vi "OOB Performance Test Channel.vi"() -> ()   [LabVIEW 2021]
uses:
  <vilib>/Platform/TimedLoop/XDataNode/timing_clust.ctl
  <vilib>/Platform/TimedLoop/XDataNode/nitl_modes.ctl
  <vilib>/Platform/TimedLoop/XDataNode/wakeup.ctl
  CIFOutOfBand.lvclass/CIFOutOfBand.ctl
  ecd22e40-9ef3-47c9-84dd-6e51471c5b7d.vi
  cc845de9-9662-4d69-8494-93190ebbf16f.vi
  5dde9a10-7574-45f3-be33-437a2b751792.vi
  630e717b-411c-4f0a-96f3-098c02e0b307.vi
  27ef35cb-55c2-4e73-bad1-dda663d636b9.vi
  ecd22e40-9ef3-47c9-84dd-6e51471c5b7d.vi/c28b0ead-42ad-4072-80a2-aca7f2bd7ce3.vi
  cc845de9-9662-4d69-8494-93190ebbf16f.vi/4bc1c15b-36ab-481f-b8dd-c64075ce723a.vi
  cc845de9-9662-4d69-8494-93190ebbf16f.vi/d83cb72b-7713-41fc-a3d1-682de79cf574.vi
  5dde9a10-7574-45f3-be33-437a2b751792.vi/c28b0ead-42ad-4072-80a2-aca7f2bd7ce3.vi
  630e717b-411c-4f0a-96f3-098c02e0b307.vi/c28b0ead-42ad-4072-80a2-aca7f2bd7ce3.vi
  630e717b-411c-4f0a-96f3-098c02e0b307.vi/219d0231-d98b-4193-b5cc-84f90e3c9091.vi
  27ef35cb-55c2-4e73-bad1-dda663d636b9.vi/c28b0ead-42ad-4072-80a2-aca7f2bd7ce3.vi
  27ef35cb-55c2-4e73-bad1-dda663d636b9.vi/219d0231-d98b-4193-b5cc-84f90e3c9091.vi
  CIF-Core-LabVIEW/src/CIFServices/CIFServices Fill In Error Info Ex.vi
  CIFOutOfBand.lvclass
  <vilib>/Platform/TimedLoop/XDataNode/XDataNode.xnode
  <vilib>/Platform/TimedLoop/XDataNode/XDNodeRunTimeDep.lvlib
  CIF-Core-LabVIEW/src/CIFServices/CifChannelServices.lvlib
panel:
  out "avg no unflat":dbl
  out "Max no unflat":dbl
  out "channel":dbl
  out "channel":dbl
  out "avg no conflict":dbl
  out "Max no conflict":dbl
  out "avg simple":dbl
  out "Max simple":dbl
  out "Max Complex":dbl
  out "avg complex":dbl
  out "pass":bool
  out "error out":errorcluster
  # "This test should be run on RT.  It stresses the communications by constantly creating resource contraints with the low priority sender and the high priority loop. On Windows the priority of the loops cannot be set."
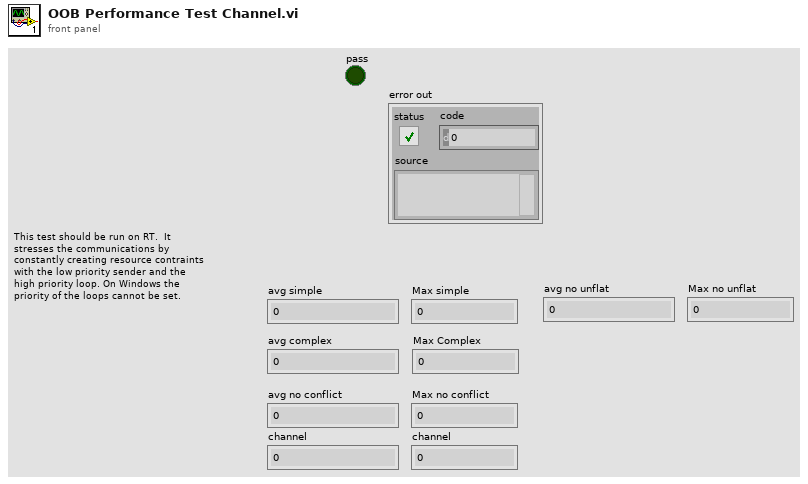
[diagram p1: front panel]
types:
  T1 = typedef "XDNodeRunTimeDep.lvlib/timing_clust.ctl" = cluster{"Expected End [f-1]":u64, "Actual End [f-1]":u64, "Finished Late? [f-1]":bool, "Expected End [i-1]":u64, "Actual End [i-1]":u64, "Finished Late? [i-1]":bool, "Expected Start [i]":u64, "Actual Start [i]":u64, "Expected Start [f]":u64, "Actual Start [f]":u64, "Source Name":string, "Structure Name":string, "Period":i64, "Deadline":i64, "Offset":i64, "Start":i64, "Priority":i32, "Timeout":i32, "Mode":T2, "Wakeup Reason":T3, "Error":errorcluster, "Source Type":string, "Secondary Source Type":string, "Global End Time":u64, "Global Start Time":u64, "Frame Duration":u64, "Iteration Duration":u64, "Assigned CPU":i32, "I/O Scan Engine Mode":u32}
  T2 = typedef "XDNodeRunTimeDep.lvlib/nitl_modes.ctl" = enum32{"No Change", "Process missed periods, maintain original phase", "Discard missed periods, maintain original phase", "Process missed periods, ignore original phase", "Discard missed periods, ignore original phase"}
  T3 = typedef "XDNodeRunTimeDep.lvlib/wakeup.ctl" = enum32{"Normal", "Aborted", "Asynchronous wakeup", "Timing source error", "Timed loop error", "Timeout"}
  T4 = cluster{"Numeric":dbl, "Array":cluster{"Numeric":dbl, "String":string, "Boolean":bool}[], "string":string, "Null array":u8[]}
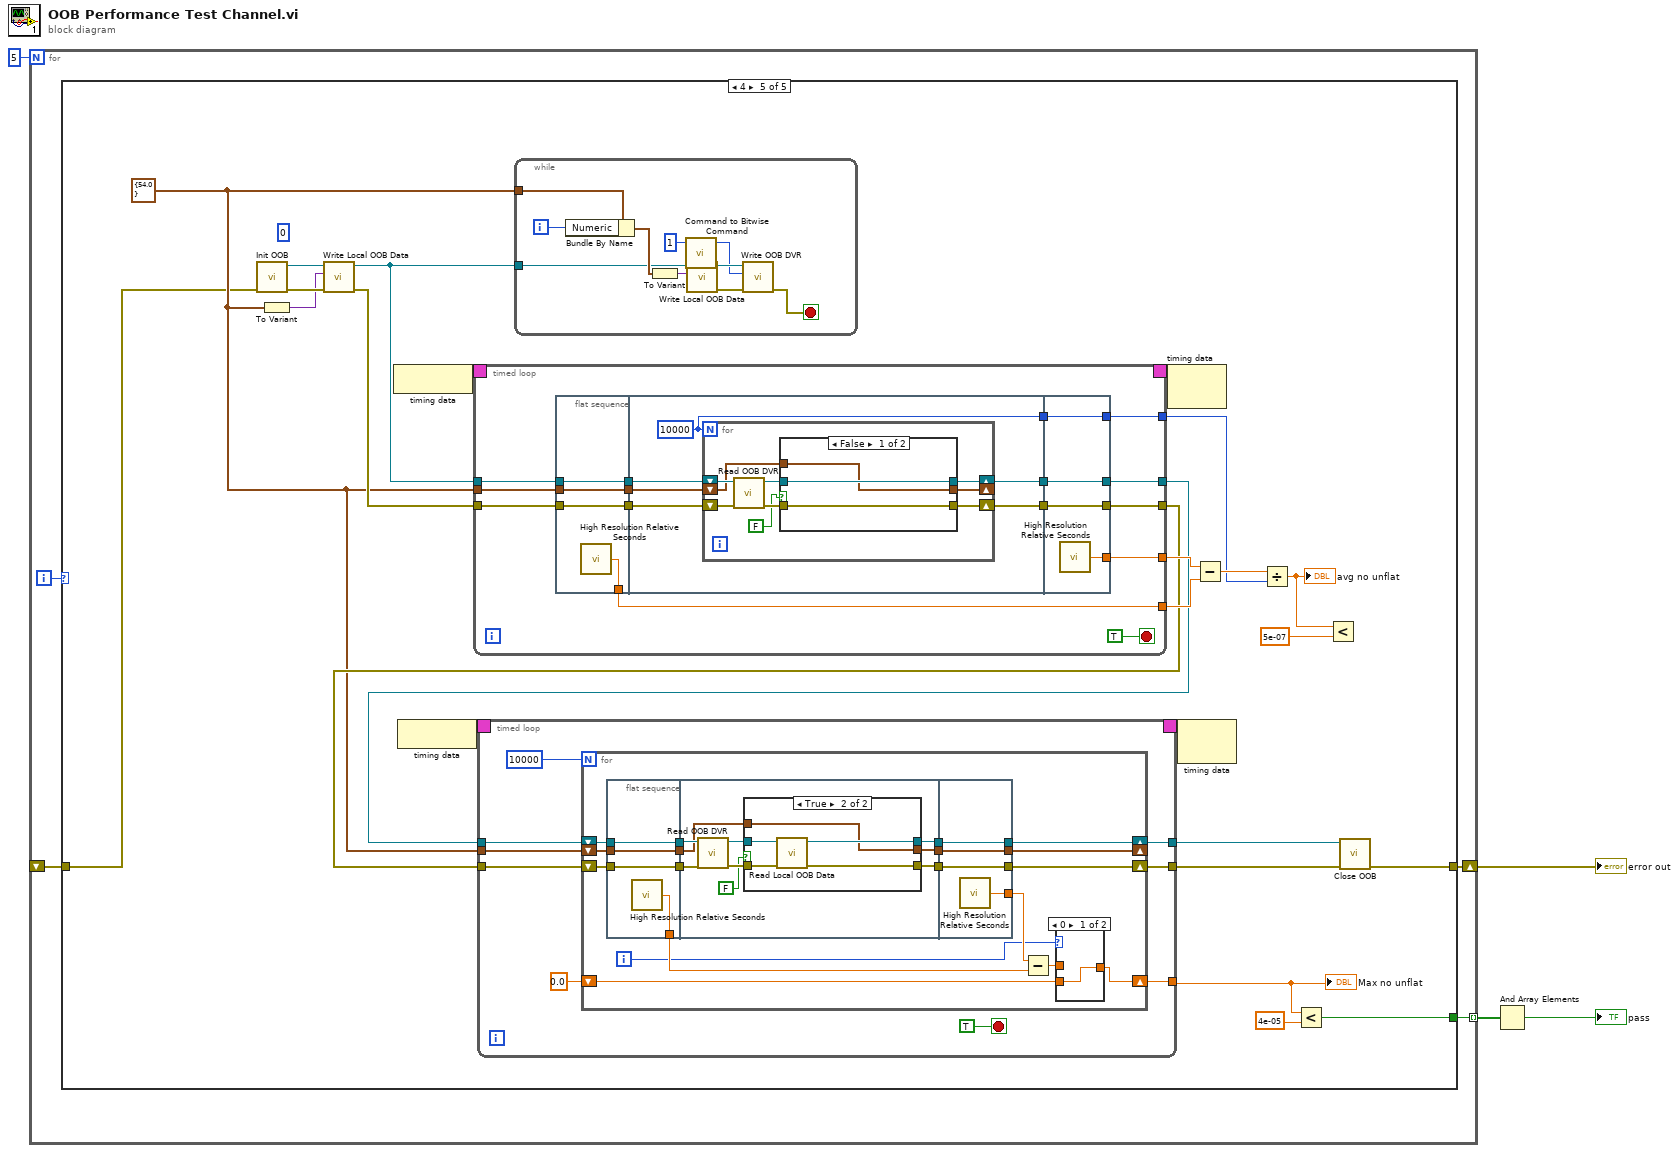
[diagram p0: block diagram]
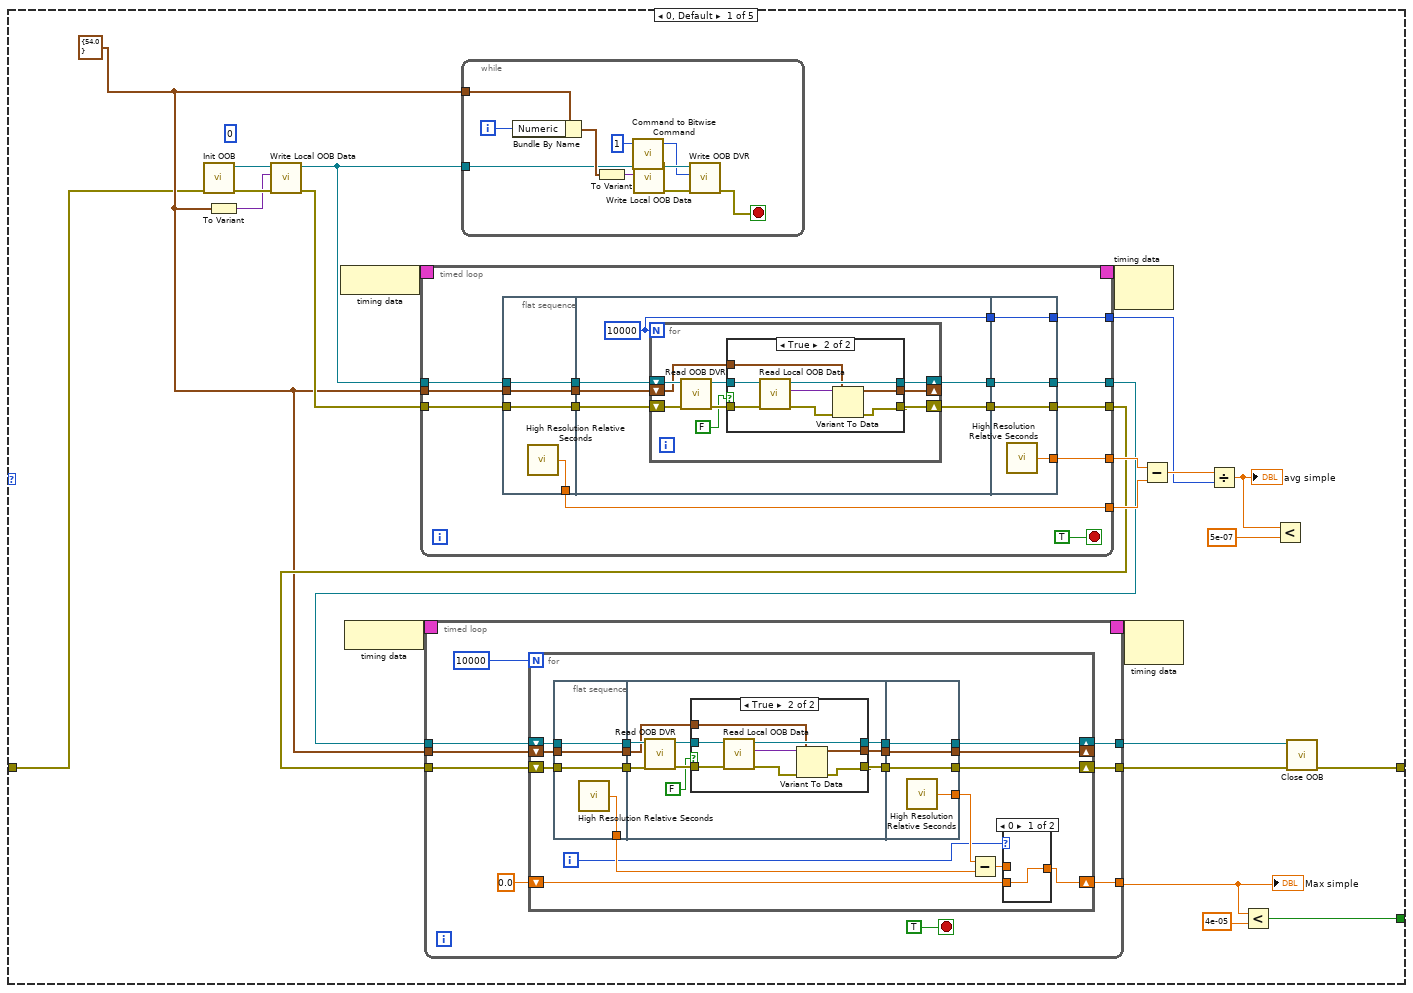
[diagram p2: hidden frame]
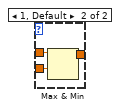
[diagram p3: hidden frame]
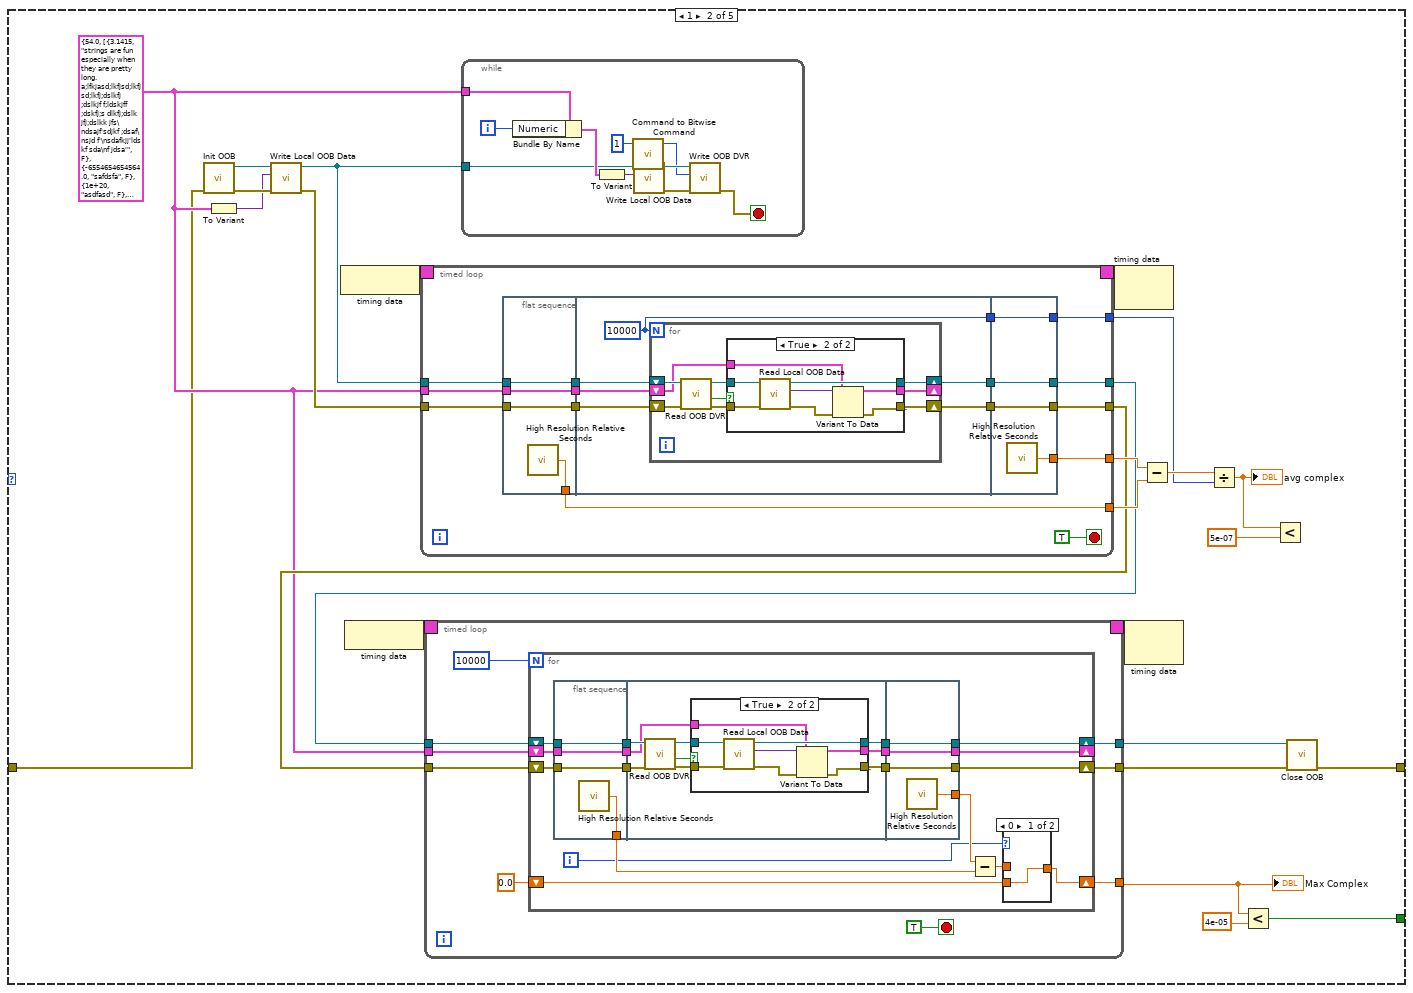
[diagram p6: hidden frame]
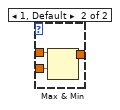
[diagram p7: hidden frame]
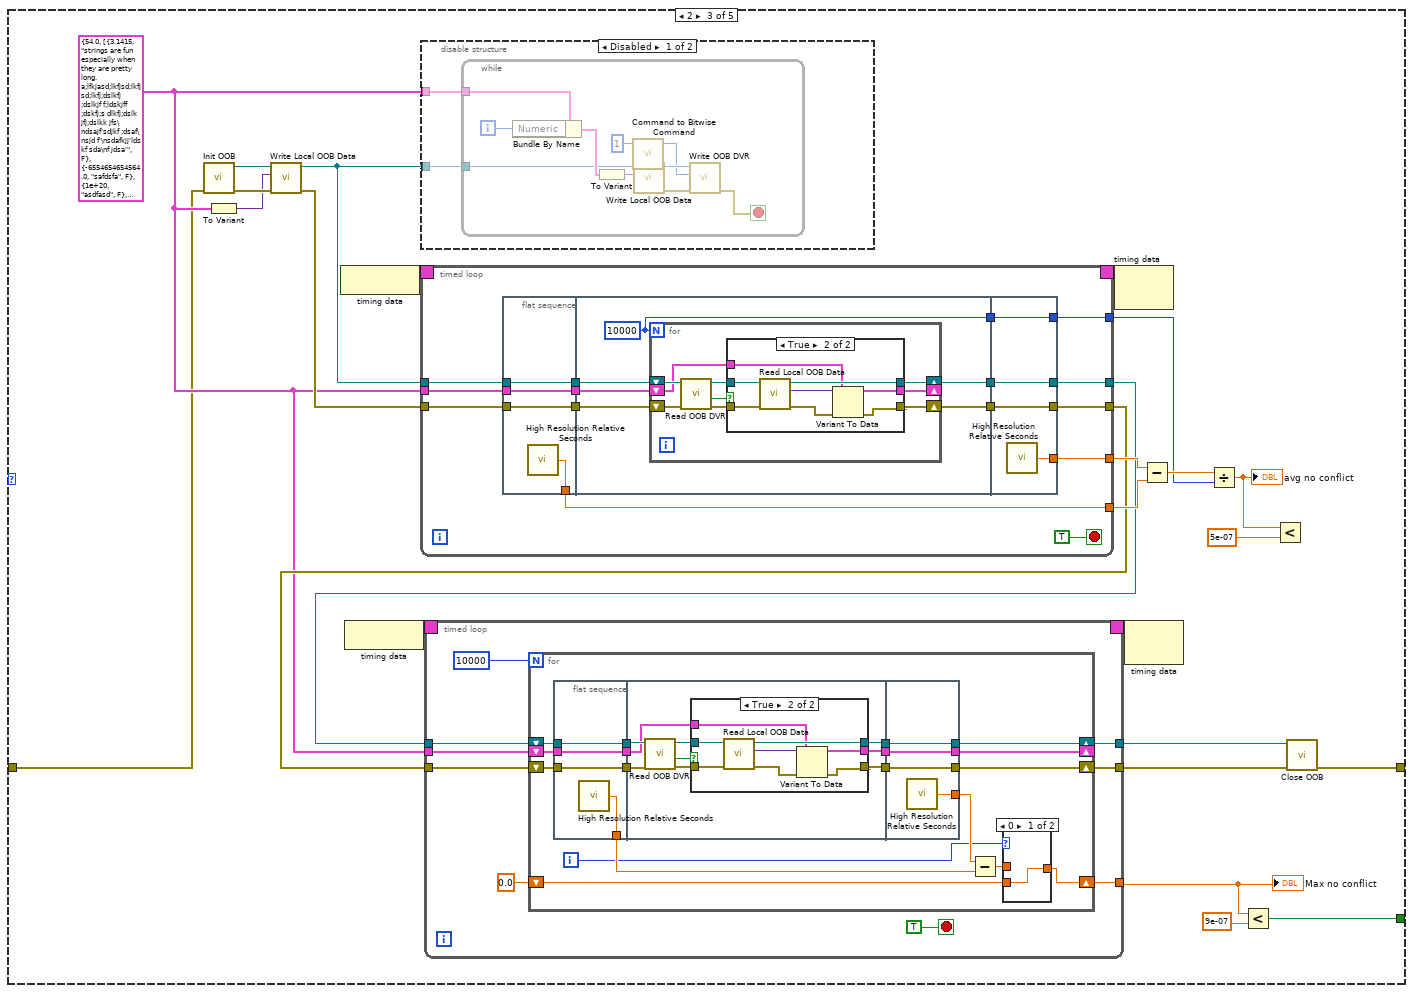
[diagram p10: hidden frame]
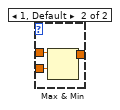
[diagram p12: hidden frame]
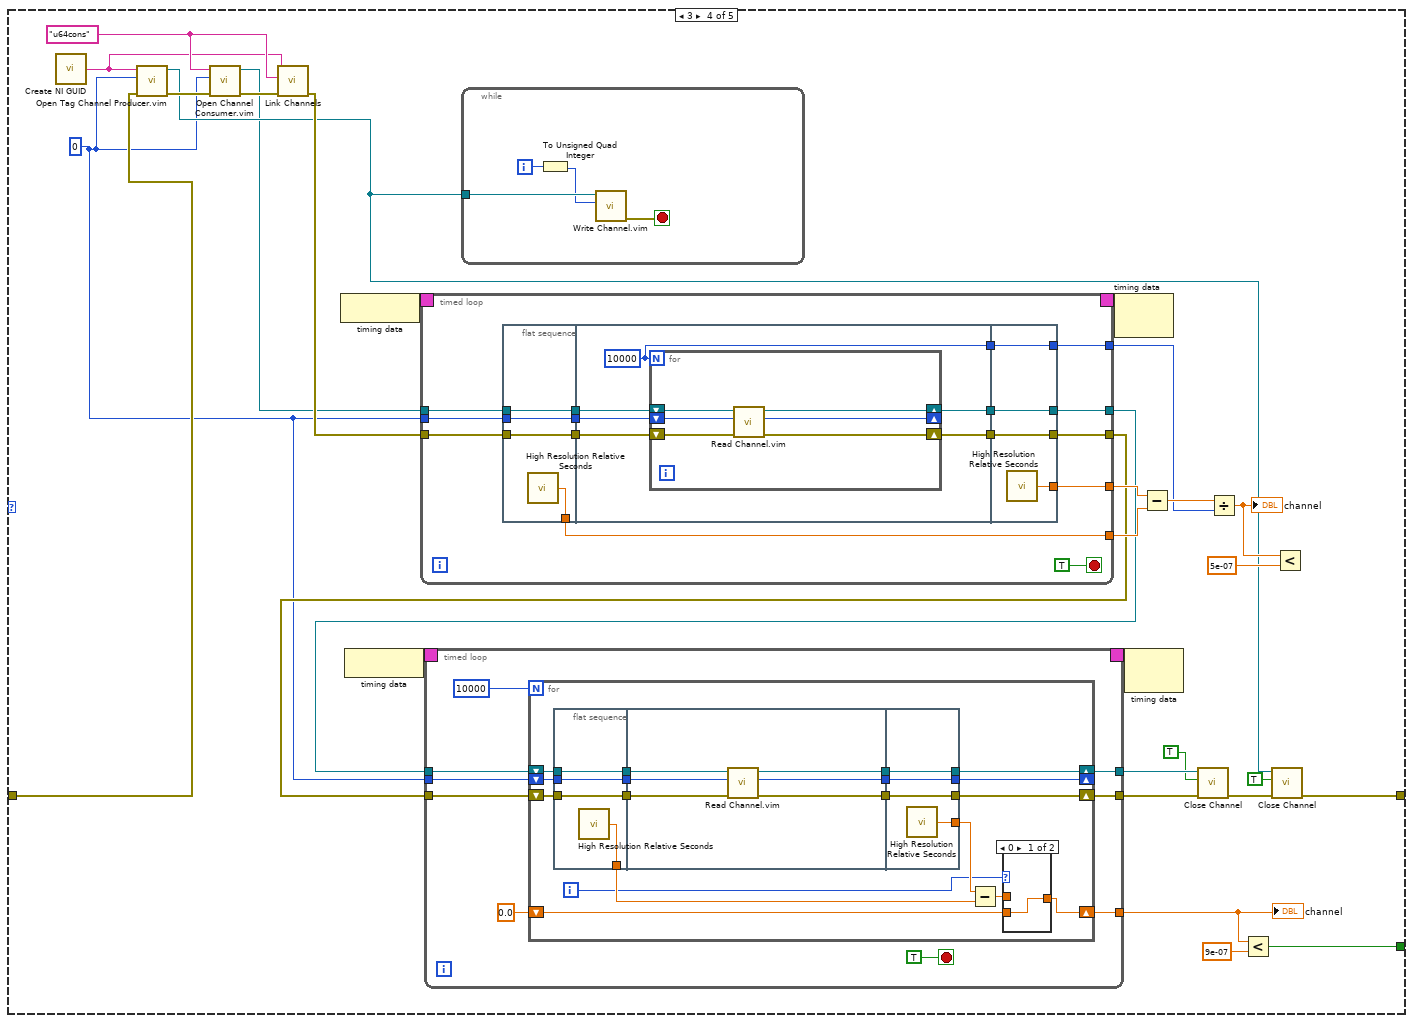
[diagram p15: hidden frame]
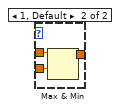
[diagram p16: hidden frame]
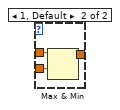
[diagram p17: hidden frame]
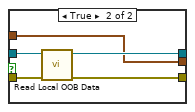
[diagram p19: hidden frame]
diagram:
  n1 = for {
    N: 5 -> [_]
    tunnel: [w8] -> w2 mode=indexing
    shift-right: [w7] -> w4
    shift-left: _ -> [w5]
    i -> [w6]
    n2 = case shown="4" w6 {
      tunnel: [w19 w168 w317 w473 w590] -> w8
      tunnel: [w16 w165 w314 w463 w587] -> w7
      tunnel: w5 -> [w9 w158 w307 w468 w580]
      frame 0, Default {
        (unwired) u64 0
        w10 = cluster{"Numeric":dbl} {"Numeric"=54.0} ("Test Config")
        n3 = call "Init OOB.vi"("error in (no error)"=w9) -> ("error out"=w15:errorcluster, "OOB out"=w13:refnum<class "CIFOutOfBand.lvclass">)  [unwired: 9 in]
        n4 = To Variant(anything=w10) -> (Variant=w14:variant)
        n5 = call "Write Local OOB Data.vi"("error in"=w15, "Local OOB Data"=w14, "OOB in"=w13) -> ("error out"=w11:errorcluster, "OOB out"=w12:refnum<class "CIFOutOfBand.lvclass">)  [unwired: 7 in]
        n6 = node-c288() -> (w33:T1)
        n7 = node-c288() -> (w31:T1)
        n8 = timed-loop {
          timing: w33 -> [_]
          timing-out: [_] -> w32
          tunnel: w12 -> [w120]
          tunnel: w11 -> [w119]
          tunnel: [w115] -> w25
          tunnel: [w113] -> w24
          tunnel: [w111] -> w29
          tunnel: [w110] -> w28
          tunnel: [w109] -> w26
          tunnel: w10 -> [w107]
          stop <- TRUE stop-if-true
          n9 = flat-sequence {
            tunnel: w119 -> [w123]
            tunnel: w120 -> [w124]
            tunnel: [w124] -> w117
            tunnel: [w123] -> w116
            tunnel: [w122] -> w110
            tunnel: w107 -> [w121]
            tunnel: [w121] -> w106
            tunnel: w117 -> [w130]
            tunnel: w116 -> [w129]
            tunnel: [w128] -> w114
            tunnel: [w127] -> w112
            tunnel: [w126] -> w108
            tunnel: w106 -> [w125]
            tunnel: [w153] -> w115
            tunnel: w114 -> [w153]
            tunnel: [w152] -> w113
            tunnel: w112 -> [w152]
            tunnel: [w151] -> w111
            tunnel: [w150] -> w109
            tunnel: w108 -> [w150]
            frame #0 {
              n10 = call <vilib>:"High Resolution Relative Seconds.vi"() -> ("relative seconds"=w122:dbl)
            }
            frame #1 {
              w126 = 10000
              n11 = for {
                N: w126 -> [_]
                shift-right: [w137] -> w128
                shift-left: w130 -> [w136]
                shift-right: [w133] -> w127
                shift-left: w129 -> [w134]
                shift-right: [w132] -> _
                shift-left: w125 -> [w135]
                n12 = call "Read OOB DVR.vi"("error in"=w134, "OOB in"=w136) -> ("error out"=w138:errorcluster, "OOB out"=w139:refnum<class "CIFOutOfBand.lvclass">)  [unwired: 6 in, 2 out]
                n13 = case shown="True" FALSE {
                  tunnel: w139 -> [w140 w149]
                  tunnel: w138 -> [w141 w148]
                  tunnel: [w140 w146] -> w137
                  tunnel: w135 -> [_ w144]
                  tunnel: [_ w142] -> w132
                  tunnel: [w141 w143] -> w133
                  frame False {
                  }
                  frame True {
                    n14 = call "Read Local OOB Data.vi"("error in"=w148, "OOB in"=w149) -> ("error out"=w147:errorcluster, "Local OOB Data"=w145:variant, "OOB out"=w146:refnum<class "CIFOutOfBand.lvclass">)  [unwired: 7 in]
                    n15 = Variant To Data(error in=w147, type=w144, Variant=w145) -> (data=w142:cluster{"Numeric":dbl}, error out=w143:errorcluster)
                  }
                }
              }
            }
            frame #2 {
              n16 = call <vilib>:"High Resolution Relative Seconds.vi"() -> ("relative seconds"=w151:dbl)
            }
          }
        }
        n17 = timed-loop {
          timing: w31 -> [_]
          timing-out: [_] -> w30
          tunnel: w25 -> [w52]
          tunnel: w24 -> [w51]
          tunnel: [w49] -> w18
          tunnel: [w48] -> w17
          tunnel: w10 -> [w47]
          tunnel: [w44] -> w21
          stop <- TRUE stop-if-true
          n18 = for {
            N: 10000 -> [_]
            shift-right: [w64] -> w49
            shift-left: w52 -> [w66]
            shift-right: [w63] -> w48
            shift-left: w51 -> [w65]
            shift-right: [w57] -> w44
            shift-left: 0.0 -> [w58]
            shift-right: [w56] -> _
            shift-left: w47 -> [w62]
            i -> [w54]
            n19 = flat-sequence {
              tunnel: w65 -> [w77]
              tunnel: w66 -> [w78]
              tunnel: [w78] -> w70
              tunnel: [w77] -> w69
              tunnel: [w76] -> w60
              tunnel: w62 -> [w75]
              tunnel: [w75] -> w68
              tunnel: w70 -> [w85]
              tunnel: w69 -> [w83]
              tunnel: [w82] -> w67
              tunnel: w68 -> [w84]
              tunnel: [w81] -> w55
              tunnel: [w80] -> w53
              tunnel: [w101] -> w64
              tunnel: w67 -> [w101]
              tunnel: [w100] -> w63
              tunnel: [w99] -> w61
              tunnel: [w98] -> w56
              tunnel: w55 -> [w98]
              tunnel: w53 -> [w100]
              frame #0 {
                n20 = call <vilib>:"High Resolution Relative Seconds.vi"() -> ("relative seconds"=w76:dbl)
              }
              frame #1 {
                n21 = call "Read OOB DVR.vi"("error in"=w83, "OOB in"=w85) -> ("error out"=w87:errorcluster, "OOB out"=w86:refnum<class "CIFOutOfBand.lvclass">)  [unwired: 6 in, 2 out]
                n22 = case shown="True" FALSE {
                  tunnel: w86 -> [w88 w97]
                  tunnel: w87 -> [w89 w96]
                  tunnel: [w88 w94] -> w82
                  tunnel: w84 -> [_ w92]
                  tunnel: [_ w90] -> w81
                  tunnel: [w89 w91] -> w80
                  frame False {
                  }
                  frame True {
                    n23 = call "Read Local OOB Data.vi"("error in"=w96, "OOB in"=w97) -> ("error out"=w95:errorcluster, "Local OOB Data"=w93:variant, "OOB out"=w94:refnum<class "CIFOutOfBand.lvclass">)  [unwired: 7 in]
                    n24 = Variant To Data(error in=w95, type=w92, Variant=w93) -> (data=w90:cluster{"Numeric":dbl}, error out=w91:errorcluster)
                  }
                }
              }
              frame #2 {
                n25 = call <vilib>:"High Resolution Relative Seconds.vi"() -> ("relative seconds"=w99:dbl)
              }
            }
            n26 = Subtract(x=w61, y=w60) -> (x-y=w59:dbl)
            n27 = case shown="0" w54 {
              tunnel: w59 -> [_ w74]
              tunnel: w58 -> [w71 w73]
              tunnel: [w71 w72] -> w57
              frame 0 {
              }
              frame 1, Default {
                n28 = Max & Min(x=w74, y=w73) -> (max(x,y)=w72:dbl)  [unwired: 1 out]
              }
            }
          }
        }
        "Max simple" <- w21
        n29 = while {
          tunnel: w12 -> [w35]
          tunnel: w10 -> [w42]
          i -> [w43]
          stop <- w34 stop-if-true
          n30 = Bundle By Name(cluster=w42, "Numeric"=w43) -> (w36:cluster{"Numeric":dbl})
          n31 = To Variant(anything=w36) -> (Variant=w38:variant)
          n32 = call "Command to Bitwise Command.vi"("OOB Command"=u8 1) -> ("bit command"=w37:u64)  [unwired: 3 in]
          n33 = call "Write Local OOB Data.vi"("Local OOB Data"=w38, "OOB in"=w35) -> ("error out"=w39:errorcluster, "OOB out"=w40:refnum<class "CIFOutOfBand.lvclass">)  [unwired: 8 in]
          n34 = call "Write OOB DVR.vi"("error in"=w39, "Commands (bitwise)"=w37, "OOB in"=w40) -> ("error out"=w34:errorcluster)  [unwired: 7 in, 1 out]
        }
        n35 = node-c288(w32) -> ()  [unwired: 1 out]
        n36 = node-c288(w30) -> ()  [unwired: 1 out]
        n37 = Subtract(x=w29, y=w28) -> (x-y=w27:dbl)
        n38 = Divide(x=w27, y=w26) -> (x/y=w23:dbl)
        "avg simple" <- w23
        n39 = Less?(x=w21, y=4e-05) -> (x < y?=w19:bool)
        n40 = Less?(x=w23, y=5e-07) -> ()  [unwired: 1 out]
        n41 = call "Close OOB.vi"("error in"=w17, "OOB in"=w18) -> ("error out"=w16:errorcluster)  [unwired: 9 in]
      }
      frame 1 {
        w159 = T4 {"Numeric"=54.0, "Array"=[{"Numeric"=3.1415, "String"="strings are fun especially when they are pretty long. a;lfkjasd;lkfjsd;lkfjsd;lkfj;dslkfj ;dslkjf f;ldskjff ;dskfj;s dlkfj;dslk jfj;dslkk jfs\ndsajf'sdjkf ;dsaf\nsjd f'\nsdafkjj'lds kf sda\nf jdsa'", "Boolean"=FALSE}, {"Numeric"=-6554654654564.0, "String"="safdsfa", "Boolean"=FALSE}, {"Numeric"=1e+20, "String"="asdfasd", "Boolean"=FALSE}, {"Numeric"=2.0, "String"="afd", "Boolean"=TRUE}, {"Numeric"=12.34, "String"="data", "Boolean"=FALSE}], "string"="strings", "Null array"=[0]} ("Test Config")
        n42 = call "Init OOB.vi"("error in (no error)"=w158) -> ("error out"=w164:errorcluster, "OOB out"=w162:refnum<class "CIFOutOfBand.lvclass">)  [unwired: 9 in]
        n43 = To Variant(anything=w159) -> (Variant=w163:variant)
        n44 = call "Write Local OOB Data.vi"("error in"=w164, "Local OOB Data"=w163, "OOB in"=w162) -> ("error out"=w160:errorcluster, "OOB out"=w161:refnum<class "CIFOutOfBand.lvclass">)  [unwired: 7 in]
        n45 = node-c288() -> (w182:T1)
        n46 = node-c288() -> (w180:T1)
        n47 = timed-loop {
          timing: w182 -> [_]
          timing-out: [_] -> w181
          tunnel: w161 -> [w269]
          tunnel: w160 -> [w268]
          tunnel: [w264] -> w174
          tunnel: [w262] -> w173
          tunnel: [w260] -> w178
          tunnel: [w259] -> w177
          tunnel: [w258] -> w175
          tunnel: w159 -> [w256]
          stop <- TRUE stop-if-true
          n48 = flat-sequence {
            tunnel: w268 -> [w272]
            tunnel: w269 -> [w273]
            tunnel: [w273] -> w266
            tunnel: [w272] -> w265
            tunnel: [w271] -> w259
            tunnel: w256 -> [w270]
            tunnel: [w270] -> w255
            tunnel: w266 -> [w279]
            tunnel: w265 -> [w278]
            tunnel: [w277] -> w263
            tunnel: [w276] -> w261
            tunnel: [w275] -> w257
            tunnel: w255 -> [w274]
            tunnel: [w302] -> w264
            tunnel: w263 -> [w302]
            tunnel: [w301] -> w262
            tunnel: w261 -> [w301]
            tunnel: [w300] -> w260
            tunnel: [w299] -> w258
            tunnel: w257 -> [w299]
            frame #0 {
              n49 = call <vilib>:"High Resolution Relative Seconds.vi"() -> ("relative seconds"=w271:dbl)
            }
            frame #1 {
              w275 = 10000
              n50 = for {
                N: w275 -> [_]
                shift-right: [w285] -> w277
                shift-left: w279 -> [w284]
                shift-right: [w281] -> w276
                shift-left: w278 -> [w282]
                shift-right: [w280] -> _
                shift-left: w274 -> [w283]
                n51 = call "Read OOB DVR.vi"("error in"=w282, "OOB in"=w284) -> ("error out"=w286:errorcluster, "New Commands"=w288:bool, "OOB out"=w287:refnum<class "CIFOutOfBand.lvclass">)  [unwired: 6 in, 1 out]
                n52 = case shown="True" w288 {
                  tunnel: w287 -> [w289 w298]
                  tunnel: w286 -> [w290 w297]
                  tunnel: [w289 w295] -> w285
                  tunnel: w283 -> [_ w293]
                  tunnel: [_ w291] -> w280
                  tunnel: [w290 w292] -> w281
                  frame False {
                  }
                  frame True {
                    n53 = call "Read Local OOB Data.vi"("error in"=w297, "OOB in"=w298) -> ("error out"=w296:errorcluster, "Local OOB Data"=w294:variant, "OOB out"=w295:refnum<class "CIFOutOfBand.lvclass">)  [unwired: 7 in]
                    n54 = Variant To Data(error in=w296, type=w293, Variant=w294) -> (data=w291:T4, error out=w292:errorcluster)
                  }
                }
              }
            }
            frame #2 {
              n55 = call <vilib>:"High Resolution Relative Seconds.vi"() -> ("relative seconds"=w300:dbl)
            }
          }
        }
        n56 = timed-loop {
          timing: w180 -> [_]
          timing-out: [_] -> w179
          tunnel: w174 -> [w201]
          tunnel: w173 -> [w200]
          tunnel: [w198] -> w167
          tunnel: [w197] -> w166
          tunnel: w159 -> [w196]
          tunnel: [w193] -> w170
          stop <- TRUE stop-if-true
          n57 = for {
            N: 10000 -> [_]
            shift-right: [w213] -> w198
            shift-left: w201 -> [w215]
            shift-right: [w212] -> w197
            shift-left: w200 -> [w214]
            shift-right: [w206] -> w193
            shift-left: 0.0 -> [w207]
            shift-right: [w205] -> _
            shift-left: w196 -> [w211]
            i -> [w203]
            n58 = flat-sequence {
              tunnel: w214 -> [w226]
              tunnel: w215 -> [w227]
              tunnel: [w227] -> w219
              tunnel: [w226] -> w218
              tunnel: [w225] -> w209
              tunnel: w211 -> [w224]
              tunnel: [w224] -> w217
              tunnel: w219 -> [w233]
              tunnel: w218 -> [w231]
              tunnel: [w230] -> w216
              tunnel: w217 -> [w232]
              tunnel: [w229] -> w204
              tunnel: [w228] -> w202
              tunnel: [w250] -> w213
              tunnel: w216 -> [w250]
              tunnel: [w249] -> w212
              tunnel: [w248] -> w210
              tunnel: [w247] -> w205
              tunnel: w204 -> [w247]
              tunnel: w202 -> [w249]
              frame #0 {
                n59 = call <vilib>:"High Resolution Relative Seconds.vi"() -> ("relative seconds"=w225:dbl)
              }
              frame #1 {
                n60 = call "Read OOB DVR.vi"("error in"=w231, "OOB in"=w233) -> ("error out"=w236:errorcluster, "New Commands"=w234:bool, "OOB out"=w235:refnum<class "CIFOutOfBand.lvclass">)  [unwired: 6 in, 1 out]
                n61 = case shown="True" w234 {
                  tunnel: w235 -> [w237 w246]
                  tunnel: w236 -> [w238 w245]
                  tunnel: [w237 w243] -> w230
                  tunnel: w232 -> [_ w241]
                  tunnel: [_ w239] -> w229
                  tunnel: [w238 w240] -> w228
                  frame False {
                  }
                  frame True {
                    n62 = call "Read Local OOB Data.vi"("error in"=w245, "OOB in"=w246) -> ("error out"=w244:errorcluster, "Local OOB Data"=w242:variant, "OOB out"=w243:refnum<class "CIFOutOfBand.lvclass">)  [unwired: 7 in]
                    n63 = Variant To Data(error in=w244, type=w241, Variant=w242) -> (data=w239:T4, error out=w240:errorcluster)
                  }
                }
              }
              frame #2 {
                n64 = call <vilib>:"High Resolution Relative Seconds.vi"() -> ("relative seconds"=w248:dbl)
              }
            }
            n65 = Subtract(x=w210, y=w209) -> (x-y=w208:dbl)
            n66 = case shown="0" w203 {
              tunnel: w208 -> [_ w223]
              tunnel: w207 -> [w220 w222]
              tunnel: [w220 w221] -> w206
              frame 0 {
              }
              frame 1, Default {
                n67 = Max & Min(x=w223, y=w222) -> (max(x,y)=w221:dbl)  [unwired: 1 out]
              }
            }
          }
        }
        "Max Complex" <- w170
        n68 = while {
          tunnel: w161 -> [w184]
          tunnel: w159 -> [w191]
          i -> [w192]
          stop <- w183 stop-if-true
          n69 = Bundle By Name(cluster=w191, "Numeric"=w192) -> (w185:T4)
          n70 = To Variant(anything=w185) -> (Variant=w187:variant)
          n71 = call "Command to Bitwise Command.vi"("OOB Command"=u8 1) -> ("bit command"=w186:u64)  [unwired: 3 in]
          n72 = call "Write Local OOB Data.vi"("Local OOB Data"=w187, "OOB in"=w184) -> ("error out"=w188:errorcluster, "OOB out"=w189:refnum<class "CIFOutOfBand.lvclass">)  [unwired: 8 in]
          n73 = call "Write OOB DVR.vi"("error in"=w188, "Commands (bitwise)"=w186, "OOB in"=w189) -> ("error out"=w183:errorcluster)  [unwired: 7 in, 1 out]
        }
        n74 = node-c288(w181) -> ()  [unwired: 1 out]
        n75 = node-c288(w179) -> ()  [unwired: 1 out]
        n76 = Subtract(x=w178, y=w177) -> (x-y=w176:dbl)
        n77 = Divide(x=w176, y=w175) -> (x/y=w172:dbl)
        "avg complex" <- w172
        n78 = Less?(x=w170, y=4e-05) -> (x < y?=w168:bool)
        n79 = Less?(x=w172, y=5e-07) -> ()  [unwired: 1 out]
        n80 = call "Close OOB.vi"("error in"=w166, "OOB in"=w167) -> ("error out"=w165:errorcluster)  [unwired: 9 in]
      }
      frame 2 {
        w308 = T4 {"Numeric"=54.0, "Array"=[{"Numeric"=3.1415, "String"="strings are fun especially when they are pretty long. a;lfkjasd;lkfjsd;lkfjsd;lkfj;dslkfj ;dslkjf f;ldskjff ;dskfj;s dlkfj;dslk jfj;dslkk jfs\ndsajf'sdjkf ;dsaf\nsjd f'\nsdafkjj'lds kf sda\nf jdsa'", "Boolean"=FALSE}, {"Numeric"=-6554654654564.0, "String"="safdsfa", "Boolean"=FALSE}, {"Numeric"=1e+20, "String"="asdfasd", "Boolean"=FALSE}, {"Numeric"=2.0, "String"="afd", "Boolean"=TRUE}, {"Numeric"=12.34, "String"="data", "Boolean"=FALSE}], "string"="strings", "Null array"=[0]} ("Test Config")
        n81 = call "Init OOB.vi"("error in (no error)"=w307) -> ("error out"=w313:errorcluster, "OOB out"=w311:refnum<class "CIFOutOfBand.lvclass">)  [unwired: 9 in]
        n82 = To Variant(anything=w308) -> (Variant=w312:variant)
        n83 = call "Write Local OOB Data.vi"("error in"=w313, "Local OOB Data"=w312, "OOB in"=w311) -> ("error out"=w309:errorcluster, "OOB out"=w310:refnum<class "CIFOutOfBand.lvclass">)  [unwired: 7 in]
        n84 = node-c288() -> (w331:T1)
        n85 = node-c288() -> (w329:T1)
        n86 = timed-loop {
          timing: w331 -> [_]
          timing-out: [_] -> w330
          tunnel: w310 -> [w420]
          tunnel: w309 -> [w419]
          tunnel: [w415] -> w323
          tunnel: [w413] -> w322
          tunnel: [w411] -> w327
          tunnel: [w410] -> w326
          tunnel: [w409] -> w324
          tunnel: w308 -> [w407]
          stop <- TRUE stop-if-true
          n87 = flat-sequence {
            tunnel: w419 -> [w423]
            tunnel: w420 -> [w424]
            tunnel: [w424] -> w417
            tunnel: [w423] -> w416
            tunnel: [w422] -> w410
            tunnel: w407 -> [w421]
            tunnel: [w421] -> w406
            tunnel: w417 -> [w430]
            tunnel: w416 -> [w429]
            tunnel: [w428] -> w414
            tunnel: [w427] -> w412
            tunnel: [w426] -> w408
            tunnel: w406 -> [w425]
            tunnel: [w453] -> w415
            tunnel: w414 -> [w453]
            tunnel: [w452] -> w413
            tunnel: w412 -> [w452]
            tunnel: [w451] -> w411
            tunnel: [w450] -> w409
            tunnel: w408 -> [w450]
            frame #0 {
              n88 = call <vilib>:"High Resolution Relative Seconds.vi"() -> ("relative seconds"=w422:dbl)
            }
            frame #1 {
              w426 = 10000
              n89 = for {
                N: w426 -> [_]
                shift-right: [w436] -> w428
                shift-left: w430 -> [w435]
                shift-right: [w432] -> w427
                shift-left: w429 -> [w433]
                shift-right: [w431] -> _
                shift-left: w425 -> [w434]
                n90 = call "Read OOB DVR.vi"("error in"=w433, "OOB in"=w435) -> ("error out"=w437:errorcluster, "New Commands"=w439:bool, "OOB out"=w438:refnum<class "CIFOutOfBand.lvclass">)  [unwired: 6 in, 1 out]
                n91 = case shown="True" w439 {
                  tunnel: w438 -> [w440 w449]
                  tunnel: w437 -> [w441 w448]
                  tunnel: [w440 w446] -> w436
                  tunnel: w434 -> [_ w444]
                  tunnel: [_ w442] -> w431
                  tunnel: [w441 w443] -> w432
                  frame False {
                  }
                  frame True {
                    n92 = call "Read Local OOB Data.vi"("error in"=w448, "OOB in"=w449) -> ("error out"=w447:errorcluster, "Local OOB Data"=w445:variant, "OOB out"=w446:refnum<class "CIFOutOfBand.lvclass">)  [unwired: 7 in]
                    n93 = Variant To Data(error in=w447, type=w444, Variant=w445) -> (data=w442:T4, error out=w443:errorcluster)
                  }
                }
              }
            }
            frame #2 {
              n94 = call <vilib>:"High Resolution Relative Seconds.vi"() -> ("relative seconds"=w451:dbl)
            }
          }
        }
        n95 = disable-structure shown="Disabled" {
          disable-tunnel: w310 -> [w333 _]
          disable-tunnel: w308 -> [w332 _]
          frame Disabled {
            n96 = while {
              tunnel: w333 -> [w335]
              tunnel: w332 -> [w342]
              i -> [w343]
              stop <- w334 stop-if-true
              n97 = Bundle By Name(cluster=w342, "Numeric"=w343) -> (w336:T4)
              n98 = To Variant(anything=w336) -> (Variant=w338:variant)
              n99 = call "Command to Bitwise Command.vi"("OOB Command"=u8 1) -> ("bit command"=w337:u64)  [unwired: 3 in]
              n100 = call "Write Local OOB Data.vi"("Local OOB Data"=w338, "OOB in"=w335) -> ("error out"=w339:errorcluster, "OOB out"=w340:refnum<class "CIFOutOfBand.lvclass">)  [unwired: 8 in]
              n101 = call "Write OOB DVR.vi"("error in"=w339, "Commands (bitwise)"=w337, "OOB in"=w340) -> ("error out"=w334:errorcluster)  [unwired: 7 in, 1 out]
            }
          }
          frame Enabled {
          }
        }
        n102 = timed-loop {
          timing: w329 -> [_]
          timing-out: [_] -> w328
          tunnel: w323 -> [w352]
          tunnel: w322 -> [w351]
          tunnel: [w349] -> w316
          tunnel: [w348] -> w315
          tunnel: w308 -> [w347]
          tunnel: [w344] -> w319
          stop <- TRUE stop-if-true
          n103 = for {
            N: 10000 -> [_]
            shift-right: [w364] -> w349
            shift-left: w352 -> [w366]
            shift-right: [w363] -> w348
            shift-left: w351 -> [w365]
            shift-right: [w357] -> w344
            shift-left: 0.0 -> [w358]
            shift-right: [w356] -> _
            shift-left: w347 -> [w362]
            i -> [w354]
            n104 = flat-sequence {
              tunnel: w365 -> [w377]
              tunnel: w366 -> [w378]
              tunnel: [w378] -> w370
              tunnel: [w377] -> w369
              tunnel: [w376] -> w360
              tunnel: w362 -> [w375]
              tunnel: [w375] -> w368
              tunnel: w370 -> [w384]
              tunnel: w369 -> [w382]
              tunnel: [w381] -> w367
              tunnel: w368 -> [w383]
              tunnel: [w380] -> w355
              tunnel: [w379] -> w353
              tunnel: [w401] -> w364
              tunnel: w367 -> [w401]
              tunnel: [w400] -> w363
              tunnel: [w399] -> w361
              tunnel: [w398] -> w356
              tunnel: w355 -> [w398]
              tunnel: w353 -> [w400]
              frame #0 {
                n105 = call <vilib>:"High Resolution Relative Seconds.vi"() -> ("relative seconds"=w376:dbl)
              }
              frame #1 {
                n106 = call "Read OOB DVR.vi"("error in"=w382, "OOB in"=w384) -> ("error out"=w387:errorcluster, "New Commands"=w385:bool, "OOB out"=w386:refnum<class "CIFOutOfBand.lvclass">)  [unwired: 6 in, 1 out]
                n107 = case shown="True" w385 {
                  tunnel: w386 -> [w388 w397]
                  tunnel: w387 -> [w389 w396]
                  tunnel: [w388 w394] -> w381
                  tunnel: w383 -> [_ w392]
                  tunnel: [_ w390] -> w380
                  tunnel: [w389 w391] -> w379
                  frame False {
                  }
                  frame True {
                    n108 = call "Read Local OOB Data.vi"("error in"=w396, "OOB in"=w397) -> ("error out"=w395:errorcluster, "Local OOB Data"=w393:variant, "OOB out"=w394:refnum<class "CIFOutOfBand.lvclass">)  [unwired: 7 in]
                    n109 = Variant To Data(error in=w395, type=w392, Variant=w393) -> (data=w390:T4, error out=w391:errorcluster)
                  }
                }
              }
              frame #2 {
                n110 = call <vilib>:"High Resolution Relative Seconds.vi"() -> ("relative seconds"=w399:dbl)
              }
            }
            n111 = Subtract(x=w361, y=w360) -> (x-y=w359:dbl)
            n112 = case shown="0" w354 {
              tunnel: w359 -> [_ w374]
              tunnel: w358 -> [w371 w373]
              tunnel: [w371 w372] -> w357
              frame 0 {
              }
              frame 1, Default {
                n113 = Max & Min(x=w374, y=w373) -> (max(x,y)=w372:dbl)  [unwired: 1 out]
              }
            }
          }
        }
        "Max no conflict" <- w319
        n114 = node-c288(w330) -> ()  [unwired: 1 out]
        n115 = node-c288(w328) -> ()  [unwired: 1 out]
        n116 = Subtract(x=w327, y=w326) -> (x-y=w325:dbl)
        n117 = Divide(x=w325, y=w324) -> (x/y=w321:dbl)
        "avg no conflict" <- w321
        n118 = Less?(x=w319, y=9e-07) -> (x < y?=w317:bool)
        n119 = Less?(x=w321, y=5e-07) -> ()  [unwired: 1 out]
        n120 = call "Close OOB.vi"("error in"=w315, "OOB in"=w316) -> ("error out"=w314:errorcluster)  [unwired: 9 in]
      }
      frame 3 {
        w470 = "u64cons" ("Channel Name")
        w458 = u64 0
        n121 = call <vilib>:"Create NI GUID.vi"() -> ("NI GUID"=w461:string)
        n122 = call "Open Tag Channel Producer.vim"("error in"=w468, "Input Type"=w458, "Channel Name"=w461) -> ("error out"=w472:errorcluster, "ADAS HIL Channel"=w462:refnum<k21>)  [unwired: 7 in]
        n123 = call "Open Channel Consumer.vim"("error in"=w472, "Input Type"=w458, "Channel Name"=w470) -> ("error out"=w471:errorcluster, "ADAS HIL Channel"=w459:refnum<k21>)  [unwired: 7 in]
        n124 = call "Link Channels.vi"("error in"=w471, "Consumer Channel Name"=w470, "Producer Channel Name"=w461) -> ("error out"=w469:errorcluster)  [unwired: 8 in]
        n125 = node-c288() -> (w487:T1)
        n126 = node-c288() -> (w485:T1)
        n127 = timed-loop {
          timing: w487 -> [_]
          timing-out: [_] -> w486
          tunnel: w459 -> [w555]
          tunnel: w469 -> [w554]
          tunnel: [w550] -> w479
          tunnel: [w548] -> w478
          tunnel: [w546] -> w483
          tunnel: [w545] -> w482
          tunnel: [w544] -> w480
          tunnel: w458 -> [w542]
          stop <- TRUE stop-if-true
          n128 = flat-sequence {
            tunnel: w554 -> [w558]
            tunnel: w555 -> [w559]
            tunnel: [w559] -> w552
            tunnel: [w558] -> w551
            tunnel: [w557] -> w545
            tunnel: w542 -> [w556]
            tunnel: [w556] -> w541
            tunnel: w552 -> [w565]
            tunnel: w551 -> [w564]
            tunnel: [w563] -> w549
            tunnel: [w562] -> w547
            tunnel: [w561] -> w543
            tunnel: w541 -> [w560]
            tunnel: [w575] -> w550
            tunnel: w549 -> [w575]
            tunnel: [w574] -> w548
            tunnel: w547 -> [w574]
            tunnel: [w573] -> w546
            tunnel: [w572] -> w544
            tunnel: w543 -> [w572]
            frame #0 {
              n129 = call <vilib>:"High Resolution Relative Seconds.vi"() -> ("relative seconds"=w557:dbl)
            }
            frame #1 {
              w561 = 10000
              n130 = for {
                N: w561 -> [_]
                shift-right: [w568] -> w563
                shift-left: w565 -> [w571]
                shift-right: [w567] -> w562
                shift-left: w564 -> [w566]
                shift-right: [w569] -> _
                shift-left: w560 -> [w570]
                n131 = call "Read Channel.vim"("error in"=w566, "Data in"=w570, "ADAS HIL Channel in"=w571) -> ("error out"=w567:errorcluster, "Data out"=w569:u64, "ADAS HIL Channel out"=w568:refnum<k21>)  [unwired: 5 in, 1 out]
              }
            }
            frame #2 {
              n132 = call <vilib>:"High Resolution Relative Seconds.vi"() -> ("relative seconds"=w573:dbl)
            }
          }
        }
        n133 = timed-loop {
          timing: w485 -> [_]
          timing-out: [_] -> w484
          tunnel: w479 -> [w500]
          tunnel: w478 -> [w499]
          tunnel: [w497] -> w466
          tunnel: [w496] -> w467
          tunnel: w458 -> [w495]
          tunnel: [w492] -> w475
          stop <- TRUE stop-if-true
          n134 = for {
            N: 10000 -> [_]
            shift-right: [w512] -> w497
            shift-left: w500 -> [w514]
            shift-right: [w511] -> w496
            shift-left: w499 -> [w513]
            shift-right: [w505] -> w492
            shift-left: 0.0 -> [w506]
            shift-right: [w504] -> _
            shift-left: w495 -> [w510]
            i -> [w502]
            n135 = flat-sequence {
              tunnel: w513 -> [w525]
              tunnel: w514 -> [w526]
              tunnel: [w526] -> w518
              tunnel: [w525] -> w517
              tunnel: [w524] -> w508
              tunnel: w510 -> [w523]
              tunnel: [w523] -> w516
              tunnel: w518 -> [w532]
              tunnel: w517 -> [w528]
              tunnel: [w531] -> w515
              tunnel: w516 -> [w530]
              tunnel: [w529] -> w503
              tunnel: [w527] -> w501
              tunnel: [w536] -> w512
              tunnel: w515 -> [w536]
              tunnel: [w535] -> w511
              tunnel: [w534] -> w509
              tunnel: [w533] -> w504
              tunnel: w503 -> [w533]
              tunnel: w501 -> [w535]
              frame #0 {
                n136 = call <vilib>:"High Resolution Relative Seconds.vi"() -> ("relative seconds"=w524:dbl)
              }
              frame #1 {
                n137 = call "Read Channel.vim"("error in"=w528, "Data in"=w530, "ADAS HIL Channel in"=w532) -> ("error out"=w527:errorcluster, "Data out"=w529:u64, "ADAS HIL Channel out"=w531:refnum<k21>)  [unwired: 5 in, 1 out]
              }
              frame #2 {
                n138 = call <vilib>:"High Resolution Relative Seconds.vi"() -> ("relative seconds"=w534:dbl)
              }
            }
            n139 = Subtract(x=w509, y=w508) -> (x-y=w507:dbl)
            n140 = case shown="0" w502 {
              tunnel: w507 -> [_ w522]
              tunnel: w506 -> [w519 w521]
              tunnel: [w519 w520] -> w505
              frame 0 {
              }
              frame 1, Default {
                n141 = Max & Min(x=w522, y=w521) -> (max(x,y)=w520:dbl)  [unwired: 1 out]
              }
            }
          }
        }
        "channel" <- w475
        n142 = while {
          tunnel: w462 -> [w490]
          i -> [w491]
          stop <- w488 stop-if-true
          n143 = To Unsigned Quad Integer(1:w491) -> (0:w489:u64)
          n144 = call "Write Channel.vim"("Data in"=w489, "ADAS HIL Channel in"=w490) -> ("error out"=w488:errorcluster)  [unwired: 7 in, 2 out]
        }
        n145 = node-c288(w486) -> ()  [unwired: 1 out]
        n146 = node-c288(w484) -> ()  [unwired: 1 out]
        n147 = Subtract(x=w483, y=w482) -> (x-y=w481:dbl)
        n148 = call "Close Channel.vi"("error in"=w467, "Force Destroy? (F)"=TRUE, "ADAS HIL Channel"=w466) -> ("error out"=w465:errorcluster)  [unwired: 8 in]
        n149 = Divide(x=w481, y=w480) -> (x/y=w477:dbl)
        "channel" <- w477
        n150 = Less?(x=w475, y=9e-07) -> (x < y?=w473:bool)
        n151 = call "Close Channel.vi"("error in"=w465, "Force Destroy? (F)"=TRUE, "ADAS HIL Channel"=w462) -> ("error out"=w463:errorcluster)  [unwired: 8 in]
        n152 = Less?(x=w477, y=5e-07) -> ()  [unwired: 1 out]
      }
      frame 4 {
        (unwired) u64 0
        w581 = cluster{"Numeric":dbl} {"Numeric"=54.0} ("Test Config")
        n153 = call "Init OOB.vi"("error in (no error)"=w580) -> ("error out"=w586:errorcluster, "OOB out"=w584:refnum<class "CIFOutOfBand.lvclass">)  [unwired: 9 in]
        n154 = To Variant(anything=w581) -> (Variant=w585:variant)
        n155 = call "Write Local OOB Data.vi"("error in"=w586, "Local OOB Data"=w585, "OOB in"=w584) -> ("error out"=w582:errorcluster, "OOB out"=w583:refnum<class "CIFOutOfBand.lvclass">)  [unwired: 7 in]
        n156 = node-c288() -> (w604:T1)
        n157 = node-c288() -> (w602:T1)
        n158 = timed-loop {
          timing: w604 -> [_]
          timing-out: [_] -> w603
          tunnel: w583 -> [w689]
          tunnel: w582 -> [w688]
          tunnel: [w684] -> w596
          tunnel: [w682] -> w595
          tunnel: [w680] -> w600
          tunnel: [w679] -> w599
          tunnel: [w678] -> w597
          tunnel: w581 -> [w676]
          stop <- TRUE stop-if-true
          n159 = flat-sequence {
            tunnel: w688 -> [w692]
            tunnel: w689 -> [w693]
            tunnel: [w693] -> w686
            tunnel: [w692] -> w685
            tunnel: [w691] -> w679
            tunnel: w676 -> [w690]
            tunnel: [w690] -> w675
            tunnel: w686 -> [w699]
            tunnel: w685 -> [w698]
            tunnel: [w697] -> w683
            tunnel: [w696] -> w681
            tunnel: [w695] -> w677
            tunnel: w675 -> [w694]
            tunnel: [w720] -> w684
            tunnel: w683 -> [w720]
            tunnel: [w719] -> w682
            tunnel: w681 -> [w719]
            tunnel: [w718] -> w680
            tunnel: [w717] -> w678
            tunnel: w677 -> [w717]
            frame #0 {
              n160 = call <vilib>:"High Resolution Relative Seconds.vi"() -> ("relative seconds"=w691:dbl)
            }
            frame #1 {
              w695 = 10000
              n161 = for {
                N: w695 -> [_]
                shift-right: [w706] -> w697
                shift-left: w699 -> [w705]
                shift-right: [w702] -> w696
                shift-left: w698 -> [w703]
                shift-right: [w701] -> _
                shift-left: w694 -> [w704]
                n162 = call "Read OOB DVR.vi"("error in"=w703, "OOB in"=w705) -> ("error out"=w707:errorcluster, "OOB out"=w708:refnum<class "CIFOutOfBand.lvclass">)  [unwired: 6 in, 2 out]
                n163 = case shown="False" FALSE {
                  tunnel: w708 -> [w710 w716]
                  tunnel: w707 -> [w711 w715]
                  tunnel: [w710 w714] -> w706
                  tunnel: w704 -> [w709 w713]
                  tunnel: [w709 w713] -> w701
                  tunnel: [w711 w712] -> w702
                  frame False {
                  }
                  frame True {
                    n164 = call "Read Local OOB Data.vi"("error in"=w715, "OOB in"=w716) -> ("error out"=w712:errorcluster, "OOB out"=w714:refnum<class "CIFOutOfBand.lvclass">)  [unwired: 7 in, 1 out]
                  }
                }
              }
            }
            frame #2 {
              n165 = call <vilib>:"High Resolution Relative Seconds.vi"() -> ("relative seconds"=w718:dbl)
            }
          }
        }
        n166 = timed-loop {
          timing: w602 -> [_]
          timing-out: [_] -> w601
          tunnel: w596 -> [w623]
          tunnel: w595 -> [w622]
          tunnel: [w620] -> w589
          tunnel: [w619] -> w588
          tunnel: w581 -> [w618]
          tunnel: [w615] -> w592
          stop <- TRUE stop-if-true
          n167 = for {
            N: 10000 -> [_]
            shift-right: [w635] -> w620
            shift-left: w623 -> [w637]
            shift-right: [w634] -> w619
            shift-left: w622 -> [w636]
            shift-right: [w628] -> w615
            shift-left: 0.0 -> [w629]
            shift-right: [w627] -> _
            shift-left: w618 -> [w633]
            i -> [w625]
            n168 = flat-sequence {
              tunnel: w636 -> [w648]
              tunnel: w637 -> [w649]
              tunnel: [w649] -> w641
              tunnel: [w648] -> w640
              tunnel: [w647] -> w631
              tunnel: w633 -> [w646]
              tunnel: [w646] -> w639
              tunnel: w641 -> [w656]
              tunnel: w640 -> [w654]
              tunnel: [w653] -> w638
              tunnel: w639 -> [w655]
              tunnel: [w652] -> w626
              tunnel: [w651] -> w624
              tunnel: [w670] -> w635
              tunnel: w638 -> [w670]
              tunnel: [w669] -> w634
              tunnel: [w668] -> w632
              tunnel: [w667] -> w627
              tunnel: w626 -> [w667]
              tunnel: w624 -> [w669]
              frame #0 {
                n169 = call <vilib>:"High Resolution Relative Seconds.vi"() -> ("relative seconds"=w647:dbl)
              }
              frame #1 {
                n170 = call "Read OOB DVR.vi"("error in"=w654, "OOB in"=w656) -> ("error out"=w658:errorcluster, "OOB out"=w657:refnum<class "CIFOutOfBand.lvclass">)  [unwired: 6 in, 2 out]
                n171 = case shown="True" FALSE {
                  tunnel: w657 -> [w660 w666]
                  tunnel: w658 -> [w661 w665]
                  tunnel: [w660 w664] -> w653
                  tunnel: w655 -> [w659 w662]
                  tunnel: [w659 w662] -> w652
                  tunnel: [w661 w663] -> w651
                  frame False {
                  }
                  frame True {
                    n172 = call "Read Local OOB Data.vi"("error in"=w665, "OOB in"=w666) -> ("error out"=w663:errorcluster, "OOB out"=w664:refnum<class "CIFOutOfBand.lvclass">)  [unwired: 7 in, 1 out]
                  }
                }
              }
              frame #2 {
                n173 = call <vilib>:"High Resolution Relative Seconds.vi"() -> ("relative seconds"=w668:dbl)
              }
            }
            n174 = Subtract(x=w632, y=w631) -> (x-y=w630:dbl)
            n175 = case shown="0" w625 {
              tunnel: w630 -> [_ w645]
              tunnel: w629 -> [w642 w644]
              tunnel: [w642 w643] -> w628
              frame 0 {
              }
              frame 1, Default {
                n176 = Max & Min(x=w645, y=w644) -> (max(x,y)=w643:dbl)  [unwired: 1 out]
              }
            }
          }
        }
        "Max no unflat" <- w592
        n177 = while {
          tunnel: w583 -> [w606]
          tunnel: w581 -> [w613]
          i -> [w614]
          stop <- w605 stop-if-true
          n178 = Bundle By Name(cluster=w613, "Numeric"=w614) -> (w607:cluster{"Numeric":dbl})
          n179 = To Variant(anything=w607) -> (Variant=w609:variant)
          n180 = call "Command to Bitwise Command.vi"("OOB Command"=u8 1) -> ("bit command"=w608:u64)  [unwired: 3 in]
          n181 = call "Write Local OOB Data.vi"("Local OOB Data"=w609, "OOB in"=w606) -> ("error out"=w610:errorcluster, "OOB out"=w611:refnum<class "CIFOutOfBand.lvclass">)  [unwired: 8 in]
          n182 = call "Write OOB DVR.vi"("error in"=w610, "Commands (bitwise)"=w608, "OOB in"=w611) -> ("error out"=w605:errorcluster)  [unwired: 7 in, 1 out]
        }
        n183 = node-c288(w603) -> ()  [unwired: 1 out]
        n184 = node-c288(w601) -> ()  [unwired: 1 out]
        n185 = Subtract(x=w600, y=w599) -> (x-y=w598:dbl)
        n186 = Divide(x=w598, y=w597) -> (x/y=w594:dbl)
        "avg no unflat" <- w594
        n187 = Less?(x=w592, y=4e-05) -> (x < y?=w590:bool)
        n188 = Less?(x=w594, y=5e-07) -> ()  [unwired: 1 out]
        n189 = call "Close OOB.vi"("error in"=w588, "OOB in"=w589) -> ("error out"=w587:errorcluster)  [unwired: 9 in]
      }
    }
  }
  "error out" <- w4
  n190 = And Array Elements(Boolean array=w2) -> (logical AND=→"pass":bool)
